vi "HIOKI PW3390 TRG.vi"(6 "OPC query (T: ON)":bool=TRUE, 8 "error in (no error)":errorcluster, 11 "VISA Resource":refnum<visa-resource-name>) -> (0 "error out":errorcluster, 3 "VISA Resource out":refnum<visa-resource-name>)   [LabVIEW 2009]
doc: "Measures once in Hold and Peak Hold status."
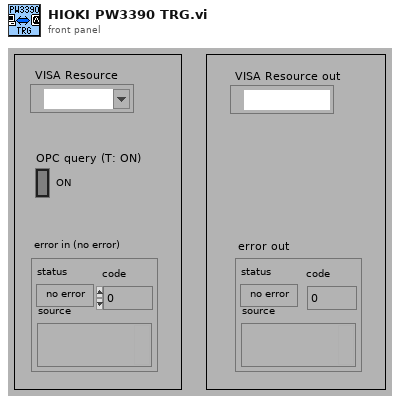
[diagram p1: front panel]
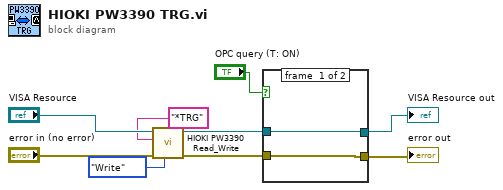
[diagram p0: block diagram]
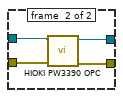
[diagram p2: hidden frame]
diagram:
  n1 = call <instrlib>:"HIOKI PW3390 Read_Write.vi"("Read/Write"=enum16{"Read", "Write"}."Write", "error in (no error)"="error in (no error)", "data in"="*TRG", "VISA Resource"="VISA Resource") -> ("error out"=w2:errorcluster, "VISA Resource out"=w3:refnum<visa-resource-name>)  [unwired: 5 in, 1 out]
  "VISA Resource out" <- w3
  n2 = case shown="TRUE" "OPC query (T: ON)" {
    tunnel: [w10 w14] -> _
    tunnel: [w9 w13] -> w1
    tunnel: w3 -> [w10 w12]
    tunnel: w2 -> [w9 w11]
    frame #0 {
    }
    frame #1 {
      n3 = call <instrlib>:"HIOKI PW3390 OPC.vi"("error in (no error)"=w11, "VISA Resource"=w12) -> ("error out"=w13:errorcluster, "VISA Resource out"=w14:refnum<visa-resource-name>)  [unwired: 7 in, 1 out]
    }
  }
  "error out" <- w1
